vi "FPGA_target_write_fifo.vi"(5 "write_FIFO":bool, 6 "mem2_addr_in":u32, 7 "mem_data_in":T1, 8 "mem2_data":u32) -> (10 "mem2_addr_dup":u32, 13 "mem_data_dup":T1, 19 "FIFO_full":bool)   [LabVIEW 2014]
doc: "writes data to internal FIFOs that used to buffer the data during pattern generation"
uses:
  FPGA_mem_data_type.ctl
  <vilib>/rvi/FIFO/Fifo_Resource/nirvififoEmulationDetermineInputValidOut.vi
  <vilib>/rvi/Emulation/niFpgaProcessEmulError.vi
  <vilib>/rvi/eio/common/nirviEmuReportErrorAndStop.vi
  <vilib>/rvi/errors/nirviReportUnexpectedCaseInternalError.vi
  <vilib>/rvi/errors/nirviReportUnexpectedCaseInternalError (U32).vi
  <vilib>/rvi/occurrence/nirviWaitOnOccurrenceBase.vi
  <vilib>/rvi/FIFO/Fifo_Resource/nirvififoEmulationReleaseLock.vi
  <vilib>/rvi/FIFO/Fifo_Resource/nirvififoEmulationObtainLock.vi
  <vilib>/rvi/FIFO/Fifo_Resource/nirvififoEmulationCreateLock.vi
  <vilib>/rvi/DataTransferAndStorage/Container/Common/niFpgaContainerGetUniqueNameForEmu.vi
  <vilib>/rvi/FIFO/Fifo_Resource/nirvififoEmulationSetSize.vi
  <vilib>/rvi/FIFO/Fifo_Resource/nirviFifoEmulationQueueMgr.vi
  <instcachedir>/0/nirviFifoEmulationQueueMgr_E5CAEC123FF24DC58D834DCA3CDAA9B5.lvgen/nirviFifoEmulationQueueMgr_E5CAEC123FF24DC58D834DCA3CDAA9B5_002.vi
  <vilib>/rvi/errors/niFpgaSetErrorForExecOnDevCompSimple.vi
  <vilib>/rvi/Emulation/niFpgaSctlEmulationGetInTimedLoop.vi
  <vilib>/rvi/Emulation/niFpgaEmulationIsFPGAContextNoSignature.vi
  <instcachedir>/0/nirviFifoEmulationQueueMgr_E5CAEC123FF24DC58D834DCA3CDAA9B5.lvgen/nirviFifoEmulationQueueMgr_E5CAEC123FF24DC58D834DCA3CDAA9B5_001.vi
  <vilib>/rvi/Emulation/niFpgaSctlEmulationResourceMgr.vi
  <vilib>/rvi/Memory/Memory_Emulation/nirvimemoryEmulationManagerCache_SetValue.vi
  <vilib>/rvi/Memory/Memory_Emulation/nirvimemoryEmulationManagerCache_GetValue.vi
  <vilib>/rvi/Memory/Memory_Emulation/nirvimemoryEmulationManagerCache_ReleaseExclusive.vi
  <vilib>/Utility/error.llb/Clear Errors.vi
  <vilib>/rvi/Memory/Memory_Emulation/nirvimemoryEmulationManagerCache_InsertValue.vi
  <vilib>/rvi/Memory/Memory_Emulation/niFpgaMemoryEmulationValidateCache.vi
  <vilib>/rvi/Memory/Memory_Emulation/nirvimemoryEmulationManagerCache_MakeExclusive.vi
  <vilib>/rvi/Memory/Memory_Emulation/niFpgaMemoryEmulationCacheClearOnFirstRun.vi
  <vilib>/rvi/Memory/Memory_Emulation/nirvimemoryEmulation.vi
  <vilib>/rvi/Memory/Memory_Emulation/nirvimemoryFastEmulation.vi
  <vilib>/rvi/DataTransferAndStorage/Container/XNode/niFpgaContainer.xnode
  <vilib>/rvi/FIFO/Fifo_Resource/nirvififoEmulationWrite.vi
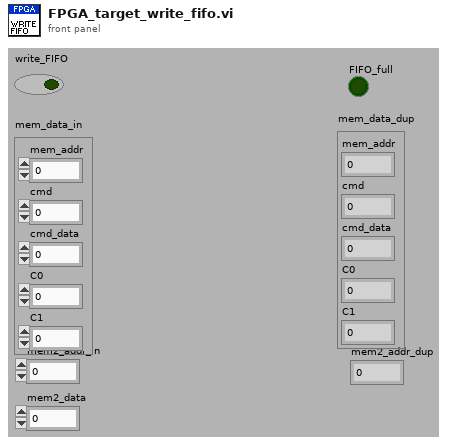
[diagram p1: front panel]
types:
  T1 = typedef "FPGA_mem_data_type.ctl" = cluster{"mem_addr":u32, "cmd":u8, "cmd_data":u32, "C0":u32, "C1":u32}
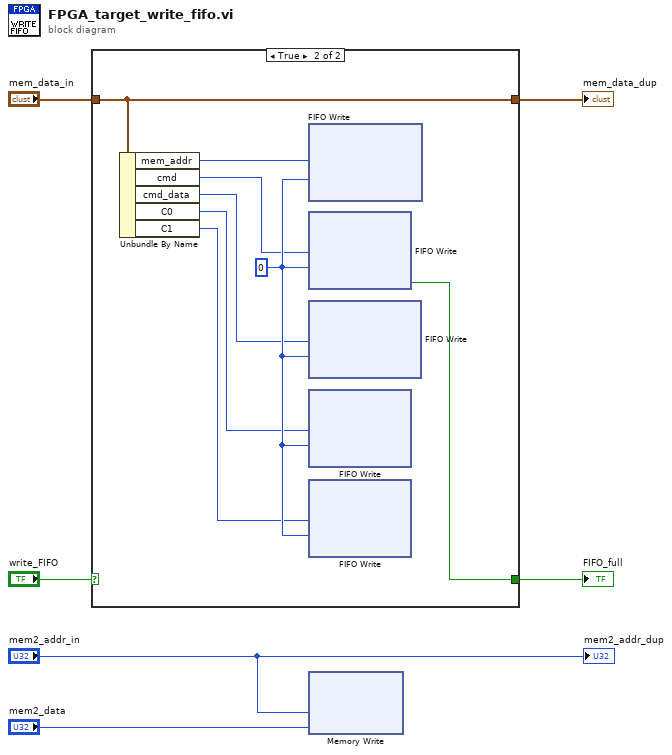
[diagram p0: block diagram]
diagram:
  n1 = case shown="True" "write_FIFO" {
    tunnel: [_ w15] -> w6
    tunnel: "mem_data_in" -> [w7 w9]
    tunnel: [w7 w9] -> w1
    frame False {
    }
    frame True {
      w14 = 0 ("Timeout")
      n2 = Unbundle By Name(w9) -> ("mem_addr"=w8:u32, "cmd"=w13:u8, "cmd_data"=w12:u32, "C0"=w11:u32, "C1"=w10:u32)
      n3 = xnode ("FIFO Write")("Element"=w8, "Timeout"=w14) -> ()  [unwired: 1 in, 2 out]
      n4 = xnode ("FIFO Write")("Element"=w13, "Timeout"=w14) -> ("Timed Out?"=w15:bool)  [unwired: 1 in, 1 out]
      n5 = xnode ("FIFO Write")("Element"=w12, "Timeout"=w14) -> ()  [unwired: 1 in, 2 out]
      n6 = xnode ("FIFO Write")("Element"=w11, "Timeout"=w14) -> ()  [unwired: 1 in, 2 out]
      n7 = xnode ("FIFO Write")("Element"=w10, "Timeout"=w14) -> ()  [unwired: 1 in, 2 out]
    }
  }
  "FIFO_full" <- w6
  "mem_data_dup" <- w1
  n8 = xnode ("Memory Write")("Address"="mem2_addr_in", "Data"="mem2_data") -> ()  [unwired: 1 in, 1 out]
  "mem2_addr_dup" <- "mem2_addr_in"
